vi "convert_to_grayscale.vi"(8 "error in (no error)":errorcluster, 11 "Image in":T2) -> (0 "error out":errorcluster, 3 "Image out":T2)   [LabVIEW 2017, in "Vision.lvlib"]
uses:
  Vision.lvlib
  <vilib>/vision/Image Controls.llb/IMAQ Image.ctl
  bin/Vision.dll
panel:
  in  "Image Type":T1 items=["Grayscale (U8)", "Grayscale (I16)", "Grayscale (SGL)", "Complex (CSG)", "RGB (U32)", "HSL (U32)", "RGB (U64)", "Grayscale (U16)"]
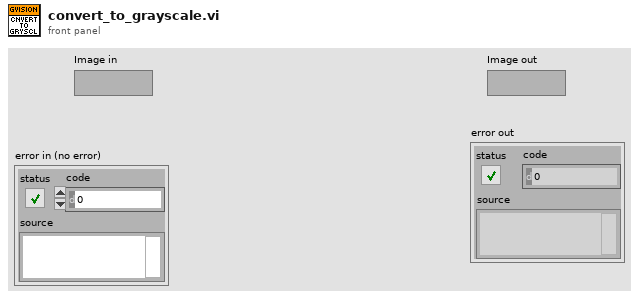
[diagram p1: front panel]
types:
  T1 = typedef "Image Type" = u32
  T2 = typedef "IMAQ Image.ctl" = refnum<image>
  T3 = enum32{"Map Pixel Pointer", "Unmap Pixel Pointer", "Get Pixels Infos"}
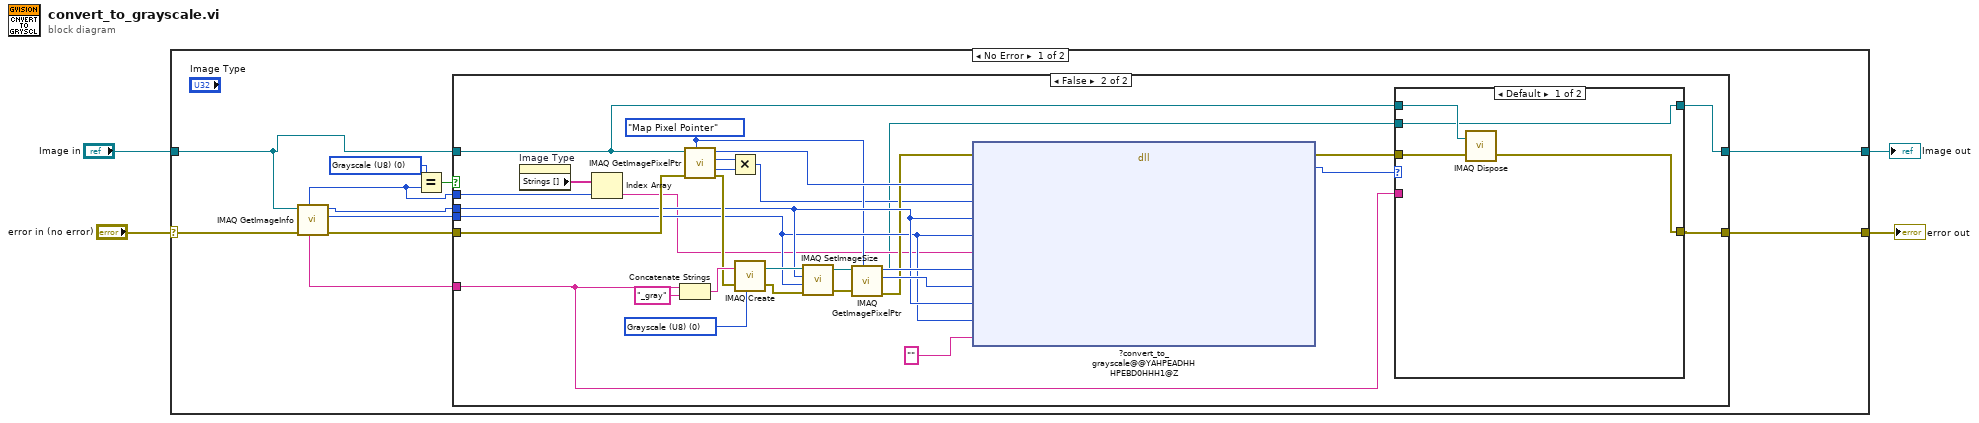
[diagram p0: block diagram]
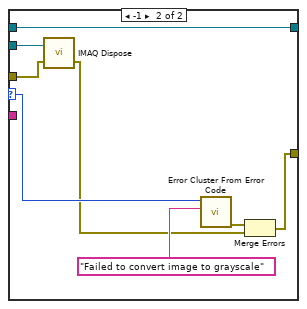
[diagram p3: hidden frame]
diagram:
  n1 = case shown="No Error" "error in (no error)" {
    selector: "error in (no error)" -> [w14 w60]
    tunnel: "Image in" -> [w10 w59]
    tunnel: [w12 w60] -> w2
    tunnel: [w11 w59] -> w1
    frame No Error {
      w5 = T1 0 items=["Grayscale (U8)", "Grayscale (I16)", "Grayscale (SGL)", "Complex (CSG)", "RGB (U32)", "HSL (U32)", "RGB (U64)", "Grayscale (U16)"] ("Image Type")
      n2 = call "IMAQ GetImageInfo"("error in (no error)"=w14, "Image"=w10) -> ("error out"=w15:errorcluster, "Y Resolution"=w7:i32, "X Resolution"=w8:i32, "Image Name"=w9:string, "Image Type"=w6:T1)  [unwired: 2 in, 3 out]
      n3 = Equal?(x=w5, y=w6) -> (x = y?=w13:bool)
      n4 = case shown="False" w13 {
        tunnel: w15 -> [w17 w44]
        tunnel: w10 -> [w16 w20]
        tunnel: [w17 w21] -> w12
        tunnel: [w16 w18] -> w11
        tunnel: w9 -> [_ w19]
        tunnel: w8 -> [_ w35]
        tunnel: w7 -> [_ w34]
        tunnel: w6 -> [_ w29]
        frame True {
        }
        frame False {
          w42 = T1 0 items=["Grayscale (U8)", "Grayscale (I16)", "Grayscale (SGL)", "Complex (CSG)", "RGB (U32)", "HSL (U32)", "RGB (U64)", "Grayscale (U16)"] ("Image Type")
          w31 = T3."Map Pixel Pointer" ("Function")
          n5 = property on="Image Type" class="Ring (strict)"() -> ("Strings []"=w30:string[])  [unwired: 2 in, 2 out]
          n6 = Index Array(array=w30, index=w29) -> (element=w28:string)
          n7 = Concatenate Strings(w19, "_gray" ("string")) -> (w45:string)
          n8 = call "IMAQ GetImagePixelPtr"("Function"=w31, "error in (no error)"=w44, "Image"=w20) -> ("error out"=w43:errorcluster, "Pixel Size (Bytes)"=w26:i32, "LineWidth(Pixels)"=w27:i32, "Pixel Pointer out"=w38:u64)  [unwired: 3 in, 2 out]
          n9 = Multiply(x=w27, y=w26) -> (x*y=w25:i32)
          n10 = call "IMAQ Create"("Image Name"=w45, "Image Type"=w42, "error in (no error)"=w43) -> ("New Image"=w41:T2, "error out"=w40:errorcluster)  [unwired: 2 in]
          n11 = call "IMAQ SetImageSize"("error in (no error)"=w40, "Y Resolution"=w34, "X Resolution"=w35, "Image"=w41) -> ("error out"=w39:errorcluster, "Image Out"=w22:T2)  [unwired: 1 in]
          n12 = call "IMAQ GetImagePixelPtr"("Function"=w31, "error in (no error)"=w39, "Image"=w22) -> ("error out"=w32:errorcluster, "LineWidth(Pixels)"=w36:i32, "Pixel Pointer out"=w37:u64)  [unwired: 3 in, 3 out]
          n13 = dll-call lib="C:/Users/Caleb/Desktop/nebraska-silicon-lab/pixel-gantry-extra/LV/bin/Vision.dll" fn="?convert_to_grayscale@@YAHPEADHHHPEBD0HHH1@Z"(error in=w32, "src_imgPtr"=w38, "src_imgLineWidth"=w25, "src_imgWidth"=w35, "src_imgHeight"=w34, "src_type"=w28, "dst_imgPtr"=w37, "dst_imgLineWidth"=w36, "dst_imgWidth"=w35, "dst_imgHeight"=w34, "log_filedir"="") -> (error out=w23:errorcluster, "return type"=w24:i32)  [unwired: 12 in, 1 out]
          n14 = case shown="Default" w24 {
            selector: w24 -> [_ w58]
            tunnel: w23 -> [w49 w52]
            tunnel: w22 -> [w48 w53]
            tunnel: [w47 w55] -> w21
            tunnel: w20 -> [w50 w54]
            tunnel: w19 -> [_ _]
            tunnel: [w48 w54] -> w18
            frame Default {
              n15 = call "IMAQ Dispose"("Image"=w50, "error in (no error)"=w49) -> ("error out"=w47:errorcluster)  [unwired: 4 in]
            }
            frame -1 {
              n16 = call "IMAQ Dispose"("Image"=w53, "error in (no error)"=w52) -> ("error out"=w51:errorcluster)  [unwired: 4 in]
              n17 = call <vilib>:"Error Cluster From Error Code.vi"("error message (\"\")"="Failed to convert image to grayscale" ("error message (\"\")"), "error code (0)"=w58) -> ("error out"=w56:errorcluster)  [unwired: 7 in]
              n18 = Merge Errors(w56, w51) -> (w55:errorcluster)
            }
          }
        }
      }
    }
    frame Error {
    }
  }
  "Image out" <- w1
  "error out" <- w2
